vi "Threshold Temp.vi"(10 "Temperature":dbl, 11 "Temp Threshold":dbl) -> (1 "Threshold Temp":bool, 2 "Auto Reset":bool, 3 "Reset":bool)   [LabVIEW 2022 SP3]
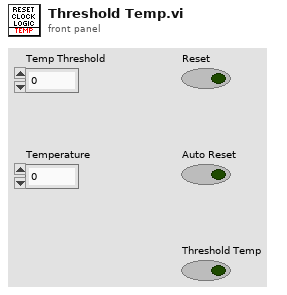
[diagram p1: front panel]
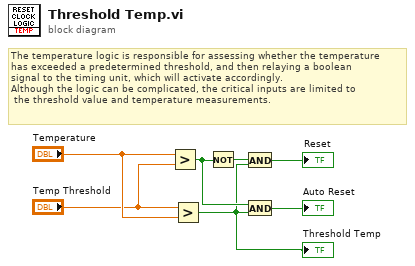
[diagram p0: block diagram]
diagram:
  # "The temperature logic is responsible for assessing whether the temperature\nhas exceeded a predetermined threshold, and then relaying a boolean \nsignal to the timing unit, which will activate accordingly. \nAlthough the logic can be complicated, the critical inputs are limited to\n the threshold value and temperature measurements."
  n1 = Greater?(x="Temperature", y="Temp Threshold") -> (0:w2:bool)
  n2 = Greater?(x="Temp Threshold", y="Temperature") -> (0:w1:bool)
  "Threshold Temp" <- w1
  n3 = Not(x=w2) -> (.not. x?=w5:bool)
  n4 = And(x=w5, y=w1) -> (x .and. y?=→"Reset":bool)
  n5 = And(x=w2, y=w1) -> (x .and. y?=→"Auto Reset":bool)
